vi "inplace_comparison.vi"() -> ()   [LabVIEW 2019]
uses:
  <vilib>/Analysis/baseanly.llb/Mean (DBL).vi
  <vilib>/Analysis/NI_AALBase.lvlib
panel:
  out "loop time 2":u32[](array[numeric])
  out "loop time 2 avg":dbl
  out "loop time 1 avg":dbl
  out "Waveform 2":waveform(dbl)
  out "Waveform":waveform(dbl)
  out "loop time 1":u32[](array[numeric])
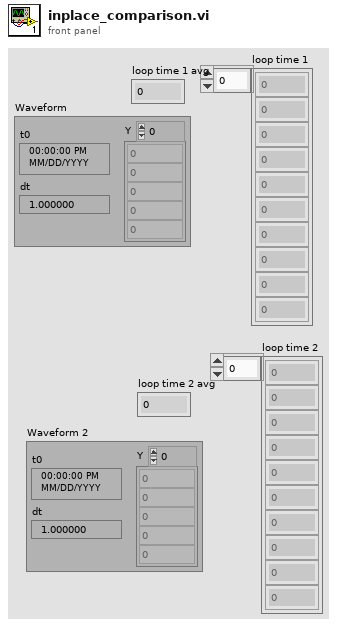
[diagram p1: front panel]
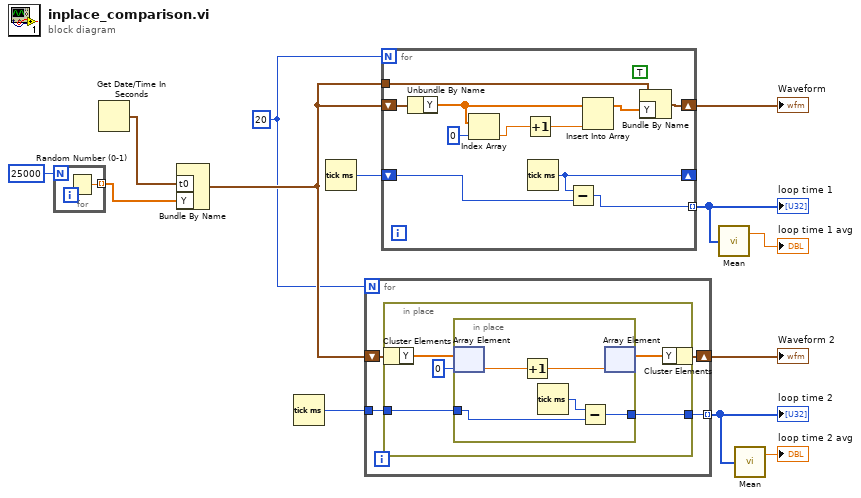
[diagram p0: block diagram]
diagram:
  w3 = 20
  n1 = for {
    N: 25000 -> [_]
    tunnel: [w14] -> w11 mode=indexing
    n2 = Random Number (0-1)() -> (number: 0 to 1=w14:dbl)
  }
  n3 = Get Date/Time In Seconds() -> (seconds since 1Jan1904=w10:timestamp)
  n4 = Bundle By Name("t0"=w10, "Y"=w11) -> (w8:waveform(dbl))  [unwired: 1 in]
  n5 = Tick Count (ms)() -> (millisecond timer value=w4:u32)
  n6 = Tick Count (ms)() -> (millisecond timer value=w12:u32)
  n7 = for {
    N: w3 -> [_]
    tunnel: w4 -> [w16]
    shift-right: [w17] -> w7
    shift-left: w8 -> [w18]
    tunnel: [w15] -> w1 mode=indexing
    n8 = in-place {
      in-place-border: w16 -> [w20]
      in-place-border: [w19] -> w15
      n9 = in-place-cluster #1(w18) -> ("Y"=w23:dbl[])
      n10 = in-place {
        in-place-border: w20 -> [w25]
        in-place-border: [w24] -> w19
        n11 = in-place-array #2(w23, 0) -> (w28:dbl)
        n12 = Increment(x=w28) -> (x+1=w27:dbl)
        n13 = Tick Count (ms)() -> (millisecond timer value=w26:u32)
        n14 = Subtract(x=w26, y=w25) -> (x-y=w24:u32)
        n15 = in-place-array #2(w27) -> (w21:dbl[])  [unwired: 1 out]
      }
      n16 = in-place-cluster #1("Y"=w21) -> (w17:waveform(dbl))
    }
  }
  "Waveform 2" <- w7
  "loop time 2" <- w1
  n17 = for {
    N: w3 -> [_]
    shift-right: [w30] -> w9
    shift-left: w8 -> [w34]
    shift-right: [w35] -> _
    shift-left: w12 -> [w36]
    tunnel: w8 -> [w31]
    tunnel: [w29] -> w6 mode=indexing
    (unwired) TRUE
    n18 = Unbundle By Name(w34) -> ("Y"=w33:dbl[])
    n19 = Index Array(array=w33, index=0) -> (element=w38:dbl)
    n20 = Increment(x=w38) -> (x+1=w37:dbl)
    n21 = Tick Count (ms)() -> (millisecond timer value=w35:u32)
    n22 = Subtract(x=w35, y=w36) -> (x-y=w29:u32)
    n23 = Insert Into Array(array=w33, new element=w37) -> (w32:dbl[])  [unwired: 1 in]
    n24 = Bundle By Name(cluster=w31, "Y"=w32) -> (w30:waveform(dbl))
  }
  "Waveform" <- w9
  "loop time 1" <- w6
  n25 = call-poly <vilib>:"Mean.vi"("X"=w6) -> ("mean"=→"loop time 1 avg":dbl)  [unwired: 1 out]
  n26 = call-poly <vilib>:"Mean.vi"("X"=w1) -> ("mean"=→"loop time 2 avg":dbl)  [unwired: 1 out]
